vi "DeviceReset.vi"(9 "Reserved":u32, 10 "DeviceInd":u32, 11 "DeviceType":u32) -> (3 "Success":bool)   [LabVIEW 2011]
uses:
  data/ControlCAN.dll
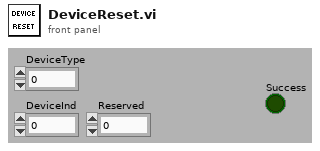
[diagram p1: front panel]
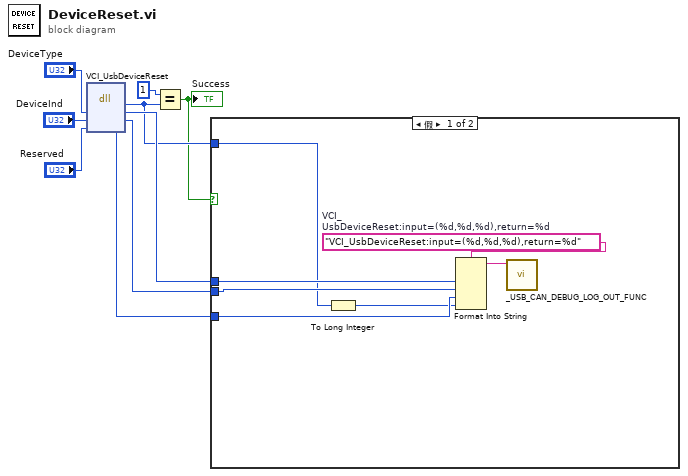
[diagram p0: block diagram]
diagram:
  n1 = dll-call lib="PTH1Mabs ZHost_E工作TnewcodeUSB CAN Tool1.97dataControlCAN.dll" fn="VCI_UsbDeviceReset" ("VCI_FindUsbDevice")("DeviceType"="DeviceType", "DeviceInd"="DeviceInd", "Reserved"="Reserved") -> ("返回类型"=w2:u32, "DeviceType"=w5:u32, "DeviceInd"=w4:u32, "Reserved"=w3:u32)  [unwired: 3 in, 2 out]
  n2 = Equal?(x=u32 1, y=w2) -> (x = y?=w1:bool)
  "Success" <- w1
  n3 = case shown="假" w1 {
    tunnel: w5 -> [w15 _]
    tunnel: w4 -> [w14 _]
    tunnel: w2 -> [w13 _]
    tunnel: w3 -> [w12 _]
    frame False {
      w10 = "VCI_UsbDeviceReset:input=(%d,%d,%d),return=%d"  # VCI_UsbDeviceReset:input=(%d,%d,%d),return=%d
      n4 = To Long Integer(number=w13) -> (32bit integer=w11:i32)
      n5 = Format Into String(format string=w10, w15, w14, w12, w11) -> (resulting string=w16:string)  [unwired: 2 in, 1 out]
      n6 = call "_USB_CAN_DEBUG_LOG_OUT_FUNC.vi"("Info"=w16) -> ()  [unwired: 11 in]
    }
    frame True {
    }
  }
